vi "Trapezoid Score 2015.vi"(10 "Rectangle Array ltrb":dbl[](array[numeric])=[2.22, 1.4], 11 "Convex Hull Area":dbl) -> (3 "Score":dbl)   [LabVIEW 2025]
doc: "Compare the area of the particle to the area of a trapezoid fit within the bounding box.\n\nPerfect trapezoid scores 100.\nLess area coverage scores lower, proportionally.\n\nExpected to be used with vision. None of the inputs are expected to be negative."
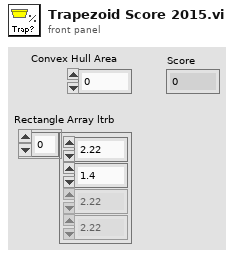
[diagram p1: front panel]
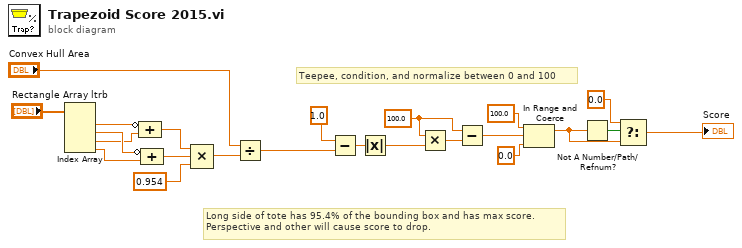
[diagram p0: block diagram]
diagram:
  w8 = 100.0 ("x/y")
  # "Teepee, condition, and normalize between 0 and 100"
  # "Long side of tote has 95.4% of the bounding box and has max score.\nPerspective and other will cause score to drop."
  n1 = Index Array(array="Rectangle Array ltrb") -> (element #1=w17:dbl, element #2=w20:dbl, element #3=w18:dbl, element #4=w19:dbl)  [unwired: 4 in]
  n2 = Compound Arithmetic op=ADD(invert w17, w18) -> (w15:dbl)
  n3 = Compound Arithmetic op=ADD(invert w20, w19) -> (w14:dbl)
  n4 = Compound Arithmetic op=MULTIPLY(w15, w14, 0.954 ("y")) -> (w21:dbl)
  n5 = Divide(x="Convex Hull Area", y=w21) -> (x/y=w5:dbl)
  n6 = Subtract(x=1.0 ("y"), y=w5) -> (x-y=w10:dbl)
  n7 = Absolute Value(x=w10) -> (abs(x)=w7:dbl)
  n8 = Multiply(x=w8, y=w7) -> (x*y=w6:dbl)
  n9 = Subtract(x=w8, y=w6) -> (x-y=w11:dbl)
  n10 = In Range and Coerce(upper limit=100.0, x=w11, lower limit=0.0) -> (coerced(x)=w2:dbl)  [unwired: 1 out]
  n11 = Not A Number/Path/Refnum?(number/path/refnum=w2) -> (NaN/Path/Refnum?=w3:bool)
  n12 = Select(t=0.0 ("y"), s=w3, f=w2) -> (s? t:f=→"Score":dbl)
